vi "adaptive filter (sub VI).vi"(0 "ERR":dbl=0.060310676968585164, 2 "輸入訊號":dbl, 3 "order":i32=10, 5 "u(收斂係數)":dbl=0.001) -> (6 "FIR輸出":dbl=-1.0516183080382016, 8 "權重":dbl[](array[numeric]))   [LabVIEW 2010]
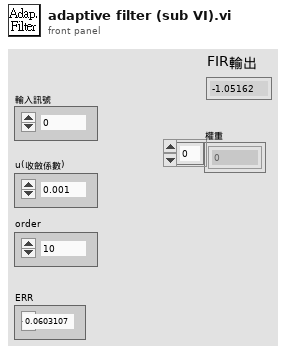
[diagram p1: front panel]
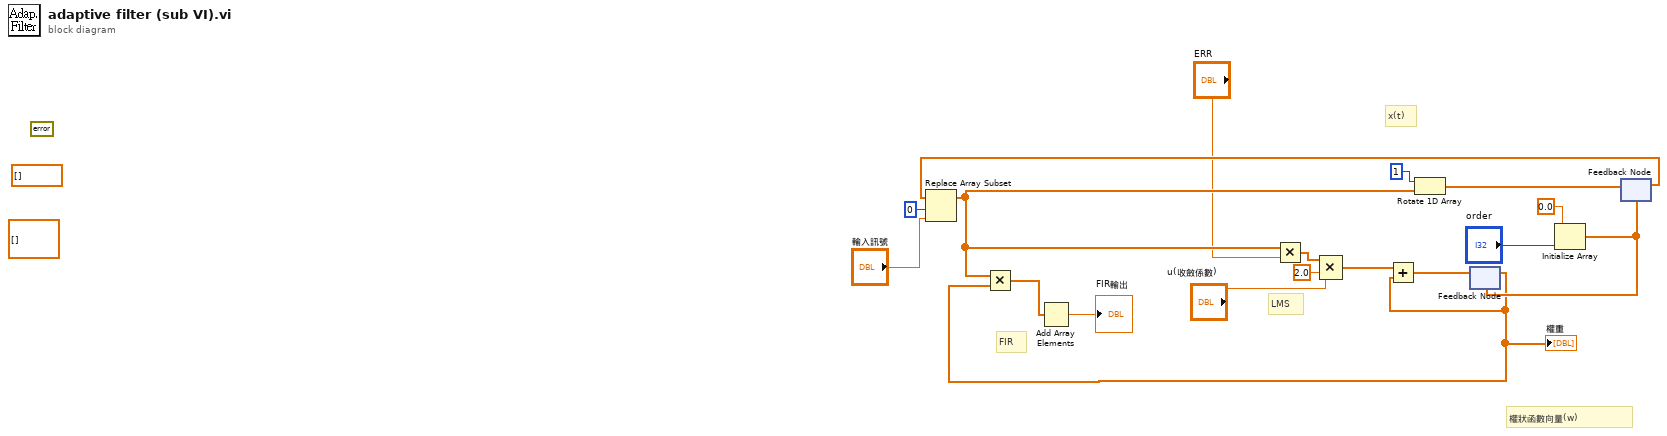
[diagram p0: block diagram]
diagram:
  (unwired) dbl[][] [] ("History Data")
  (unwired) dbl[] [] ("History Data")
  (unwired) errorcluster {"status"=FALSE, "code"=0, "source"=""} ("error constant")
  # "LMS"
  # "FIR"
  # "權狀函數向量(w)"
  # "x(t)"
  n1 = Initialize Array(0.0 ("element"), "order") -> (w3:dbl[])
  n2 = feedback #1(w3) -> (w1:dbl[])
  "權重" <- w1
  n3 = feedback #2(w3) -> (w8:dbl[])
  n4 = Replace Array Subset(array=w8, new element="輸入訊號", index=0) -> (w13:dbl[])
  n5 = Multiply(x=w13, y=w1) -> (x*y=w11:dbl[])
  n6 = Add Array Elements(numeric array=w11) -> (sum=→"FIR輸出":dbl)
  n7 = Multiply(x=w13, y="ERR") -> (x*y=w18:dbl[])
  n8 = Compound Arithmetic op=MULTIPLY(w18, 2.0 ("value"), "u(收斂係數)") -> (w4:dbl[])
  n9 = Add(x=w4, y=w1) -> (x+y=w5:dbl[])
  n10 = Rotate 1D Array(1:w13, 2:1 ("n")) -> (0:w9:dbl[])
  n11 = feedback-in #1(w5) -> ()
  n12 = feedback-in #2(w9) -> ()
